vi "write_exp_event.vi"() -> ()   [LabVIEW 2013]
uses:
  Controls/Slave Loop Cases/slave_cases.ctl
panel:
  out "error out":errorcluster
  in  "error in (no error)":errorcluster
  in  "Queue Element":cluster{T1, "variant":variant}={enum."Idle", "variant"=variant}
  in  "Q ref In":refnum<queue>
  out "Q ref Out":refnum<queue>
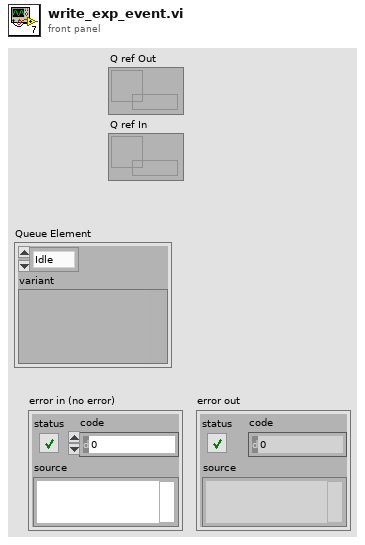
[diagram p1: front panel]
types:
  T1 = typedef "slave_cases.ctl" = enum16{"Initialize", "Idle", "Gen Scan Array", "Write Experiment", "Write Batch File", "Wait For Data", "Analyze and Display Data", "Scan Parameters", "Save Data", "Error", "Shutdown"}
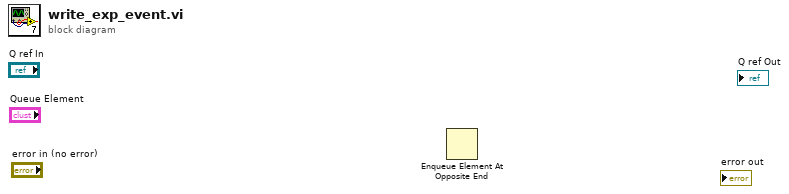
[diagram p0: block diagram]
diagram:
  n1 = Enqueue Element At Opposite End() -> ()  [unwired: 4 in, 3 out]
